vi "Log_Q Ref.vi"(3 "Close":bool) -> (1 "Log Queue":refnum<queue>)   [LabVIEW 2015]
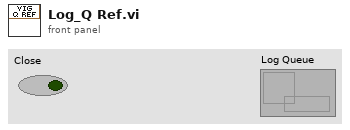
[diagram p1: front panel]
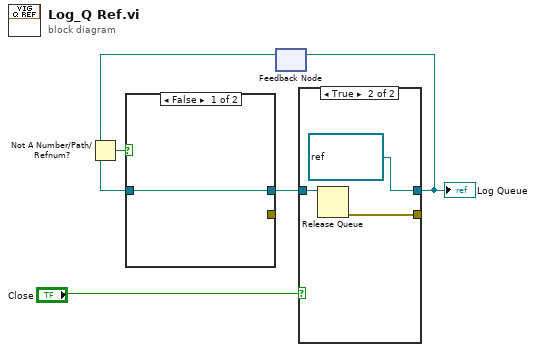
[diagram p0: block diagram]
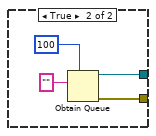
[diagram p3: hidden frame]
diagram:
  n1 = feedback #1() -> (w4:refnum<queue>)  [unwired: 1 in]
  n2 = Not A Number/Path/Refnum?(number/path/refnum=w4) -> (NaN/Path/Refnum?=w5:bool)
  n3 = case shown="False" w5 {
    tunnel: [w6 w9] -> w3
    tunnel: w4 -> [w6 _]
    tunnel: [_ w8] -> _
    frame False {
    }
    frame True {
      n4 = Obtain Queue(max queue size (-1, unlimited)=100, element data type="") -> (queue out=w9:refnum<queue>, error out=w8:errorcluster)  [unwired: 3 in, 1 out]
    }
  }
  n5 = case shown="True" "Close" {
    tunnel: w3 -> [w11 w14]
    tunnel: [w11 refnum<queue> refnum ("queue out")] -> w2
    tunnel: [_ w13] -> _
    frame False {
    }
    frame True {
      n6 = Release Queue(queue=w14) -> (error out=w13:errorcluster)  [unwired: 2 in, 2 out]
    }
  }
  "Log Queue" <- w2
  n7 = feedback-in #1(w2) -> ()
